vi "Tolerance.vi"(9 "Setpoint":dbl, 10 "Tolerance":dbl, 11 "Current Value":dbl) -> (3 "In Range?":bool)   [LabVIEW 2016]
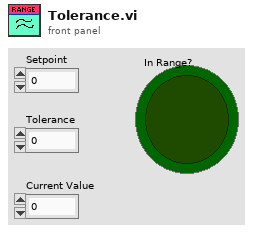
[diagram p1: front panel]
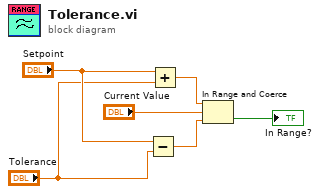
[diagram p0: block diagram]
diagram:
  n1 = Subtract(x="Setpoint", y="Tolerance") -> (x-y=w4:dbl)
  n2 = Add(x="Setpoint", y="Tolerance") -> (x+y=w5:dbl)
  n3 = In Range and Coerce(upper limit=w5, x="Current Value", lower limit=w4) -> (In Range?=→"In Range?":bool)  [unwired: 1 out]
